vi "GOOPUtil Demo.vi"() -> ()   [LabVIEW 2012]
uses:
  <vilib>/addons/GOOPUtility/GOOPUtil_MemberDefinition.ctl
  <vilib>/addons/GOOPUtility/_Demo/GOOPUtil_Demo/AnotherClass_class/AnotherClass.lvclass
  <vilib>/addons/GOOPUtility/_Demo/GOOPUtil_Demo/DemoClass1_class/DemoClass1.lvclass
  <vilib>/addons/GOOPUtility/_Demo/GOOPUtil_Demo/DemoSubClass1_class/DemoSubClass1.lvclass
  <vilib>/addons/GOOPUtility/_Demo/GOOPUtil_Demo/DemoSubClass2_class/DemoSubClass2.lvclass
  <vilib>/addons/GOOPUtility/_Demo/GOOPUtil_Demo/DemoSubSubClass1_class/DemoSubSubClass1.lvclass
  <vilib>/addons/GOOPUtility/GOOPUtility.lvlib
panel:
  out "Class Path":path
  out "Another class constant IsEmpty?":bool
  out "AnotherClass constant Not a refnum?":bool
  out "Another Class Not a refnum?":bool
  out "Has AnotherClass SameAncestor DemoSubClass2?":bool
  out "Has DemoSubSubClass 1 SameAncestor DemoSubClass2?":bool
  out "Is DemoSubClass1 InstanceOf DemoSubClass2":bool
  out "Is DemoSubSubClass 1 InstanceOf DemoSubClass1?":bool
  out "Full Class Name":string
  out "lvlib Hierarchy":string[](array[string])
  out "Class Name":string
  out "IsCastReferenceEmpty?":bool
  out "IsLVObjectEmpty?":bool
  out "MemberPaths":T1[](array[typedef])
  out "Nr Of Killed Objects":i32
  out "error out":errorcluster
  in  "Destructor":enum16{"Generic Destroy", "Garbage Collector"}(ring)
  # "1. LV Object constant"
  # "2. DemoClass1 object"
  # "Doesn't work when\n.lvclass is inside an exe."
  # "3. DemoSubClass1 object"
  # "4. DemoSubSubClass object"
  # "5. DemoSubClass1 object"
  # "6. AnotherClass object"
  # "Notice: When building an application, the front panels of the Create(), Destroy() and GetObjectStatus()\nmustn't be removed. There is a trick to prevent them to be removed, by adding a \"dummy\"\ncontrol reference (or local variable) to the diagram somewhere, else you have to change the\nsettings in the build script for each of these VIs."
  # "7. AnotherClass constant"
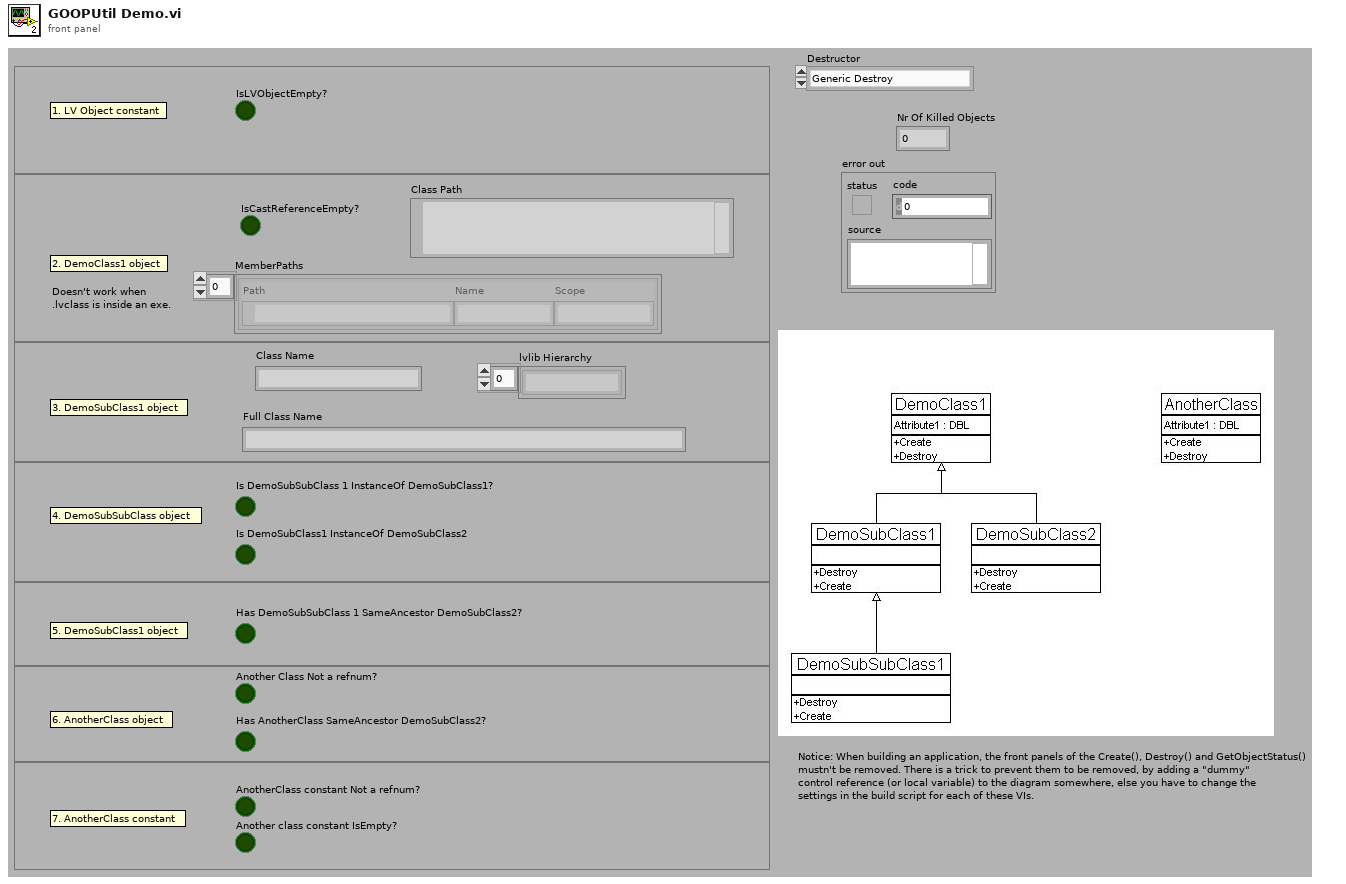
[diagram p1: front panel]
types:
  T1 = typedef "GOOPUtility.lvlib/GOOPUtil_MemberDefinition.ctl" = cluster{"Path":path, "Name":string, "Scope":string}
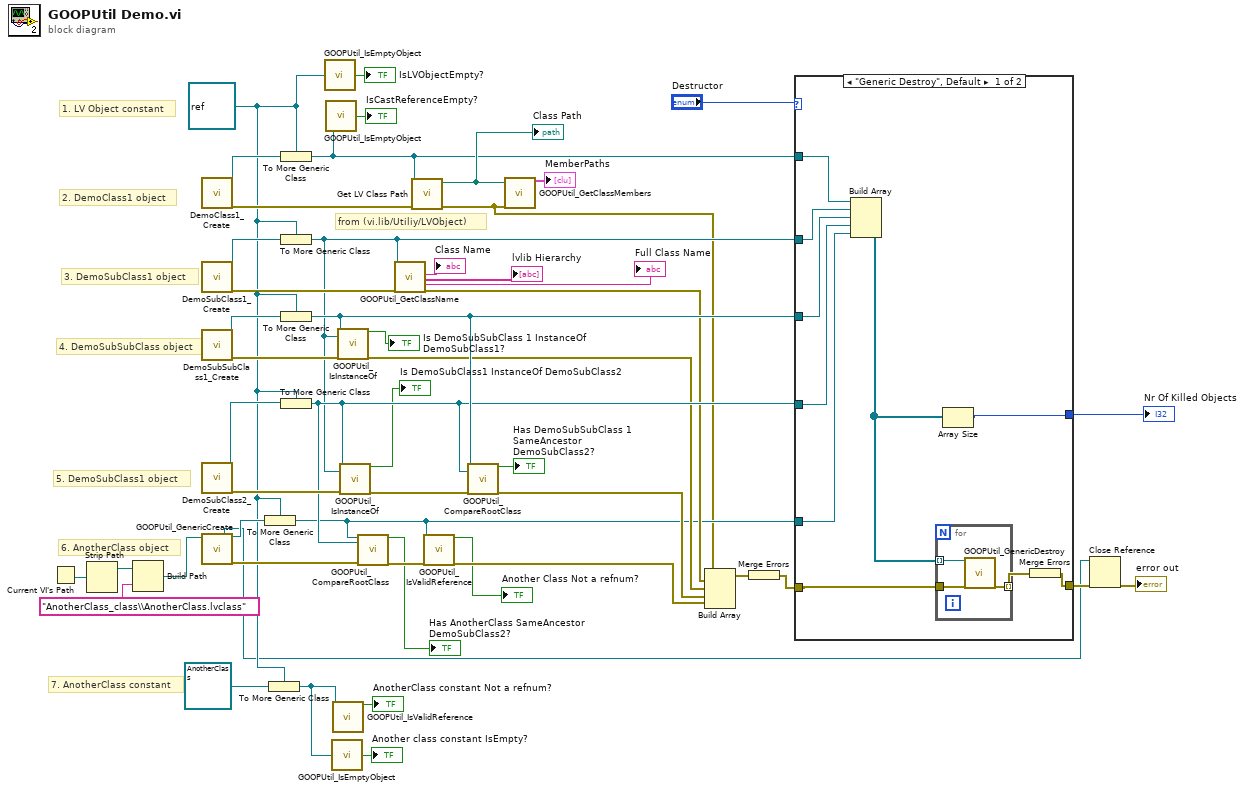
[diagram p0: block diagram]
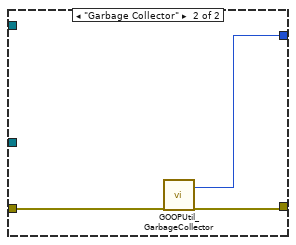
[diagram p2: hidden frame]
diagram:
  w26 = refnum<class> refnum ("LabVIEW Object")
  # "7. AnotherClass constant"
  # "6. AnotherClass object"
  # "5. DemoSubClass1 object"
  # "4. DemoSubSubClass object"
  # "3. DemoSubClass1 object"
  # "2. DemoClass1 object"
  # "1. LV Object constant"
  # "from (vi.lib/Utiliy/LVObject)"
  n1 = Current VI's Path() -> (path=w7:path)
  n2 = Strip Path(path=w7) -> (stripped path=w6:path)  [unwired: 1 out]
  n3 = Build Path(base path=w6, name or relative path="AnotherClass_class\\AnotherClass.lvclass") -> (appended path=w5:path)
  n4 = call <vilib>:"DemoClass1_Create.vi"() -> ("reference out"=w49:refnum<class "DemoClass1.lvclass">, "error out"=w41:errorcluster)  [unwired: 18 in]
  n5 = call <vilib>:"DemoSubClass1_Create.vi"() -> ("reference out"=w48:refnum<class "DemoSubClass1.lvclass">, "error out"=w32:errorcluster)  [unwired: 18 in]
  n6 = call <vilib>:"DemoSubSubClass1_Create.vi"() -> ("reference out"=w47:refnum<class "DemoSubSubClass1.lvclass">, "error out"=w37:errorcluster)  [unwired: 18 in]
  n7 = call <vilib>:"DemoSubClass2_Create.vi"() -> ("reference out"=w46:refnum<class "DemoSubClass2.lvclass">, "error out"=w38:errorcluster)  [unwired: 18 in]
  n8 = call <vilib>:"GOOPUtil_GenericCreate.vi"("GOOP Class Path"=w5) -> ("GOOP constructor VI ref"=w1:refnum<vi>, "GOOP Object"=w45:refnum<class>, "error out"=w36:errorcluster)  [unwired: 16 in]
  n9 = To More Generic Class(target class=w26, reference=w45) -> (generic class reference=w20:refnum<class>)
  n10 = To More Generic Class(target class=w26, reference=refnum<class "AnotherClass.lvclass"> refnum ("reference out")) -> (generic class reference=w21:refnum<class>)
  n11 = To More Generic Class(target class=w26, reference=w49) -> (generic class reference=w28:refnum<class>)
  n12 = To More Generic Class(target class=w26, reference=w48) -> (generic class reference=w30:refnum<class>)
  n13 = To More Generic Class(target class=w26, reference=w47) -> (generic class reference=w34:refnum<class>)
  n14 = To More Generic Class(target class=w26, reference=w46) -> (generic class reference=w33:refnum<class>)
  n15 = call <vilib>:"GOOPUtil_IsEmptyObject.vi"("LabVIEW Object"=w26) -> ("IsEmpty?"=→"IsLVObjectEmpty?":bool)
  n16 = call <vilib>:"GOOPUtil_IsEmptyObject.vi"("LabVIEW Object"=w28) -> ("IsEmpty?"=→"IsCastReferenceEmpty?":bool)
  n17 = call <vilib>:"GOOPUtil_IsEmptyObject.vi"("LabVIEW Object"=w21) -> ("IsEmpty?"=→"Another class constant IsEmpty?":bool)
  n18 = call <vilib>:"GOOPUtil_IsValidReference.vi"("LabVIEW Object"=w21) -> ("Not a refnum?"=→"AnotherClass constant Not a refnum?":bool)  [unwired: 16 in, 2 out]
  n19 = call <vilib>:"GOOPUtil_IsInstanceOf.vi"("GOOP Object"=w34, "Is Instance of Object"=w30, "error in (no error)"=w37) -> ("IsInstanceOf"=→"Is DemoSubSubClass 1 InstanceOf DemoSubClass1?":bool, "error out"=w24:errorcluster)  [unwired: 15 in]
  n20 = call <vilib>:"GOOPUtil_IsInstanceOf.vi"("GOOP Object"=w33, "Is Instance of Object"=w30, "error in (no error)"=w38) -> ("IsInstanceOf"=→"Is DemoSubClass1 InstanceOf DemoSubClass2":bool, "error out"=w35:errorcluster)  [unwired: 15 in]
  n21 = call <vilib>:"GOOPUtil_CompareRootClass.vi"("GOOP Object 1"=w20, "GOOP Object 2"=w33, "error in (no error)"=w36) -> ("SameAncestor"=→"Has AnotherClass SameAncestor DemoSubClass2?":bool, "error out"=w25:errorcluster)  [unwired: 13 in, 2 out]
  n22 = call <vilib>:"GOOPUtil_GetClassName.vi"("LabVIEW Object"=w30, "error in (no error)"=w32) -> ("Class Name"=→"Class Name":string, "lvlib Hierarchy"=→"lvlib Hierarchy":string[], "Full Class Name"=→"Full Class Name":string, "error out"=w31:errorcluster)  [unwired: 13 in, 1 out]
  n23 = call <vilib>:"Get LV Class Path.vi"("error in (no error)"=w41, "object"=w28) -> ("error out"=w8:errorcluster, "class path"=w40:path)  [unwired: 8 in]
  "Class Path" <- w40
  n24 = call <vilib>:"GOOPUtil_IsValidReference.vi"("LabVIEW Object"=w20, "error in (no error)"=w25) -> ("Not a refnum?"=→"Another Class Not a refnum?":bool, "error out"=w22:errorcluster)  [unwired: 15 in, 1 out]
  n25 = call <vilib>:"GOOPUtil_CompareRootClass.vi"("GOOP Object 1"=w34, "GOOP Object 2"=w33, "error in (no error)"=w35) -> ("SameAncestor"=→"Has DemoSubSubClass 1 SameAncestor DemoSubClass2?":bool, "error out"=w23:errorcluster)  [unwired: 13 in, 2 out]
  n26 = call <vilib>:"GOOPUtil_GetClassMembers.vi"("LVClassPath"=w40, "error in (no error)"=w8) -> ("MemberPaths"=→"MemberPaths":T1[])  [unwired: 16 in, 1 out]
  n27 = Build Array(w8, w31, w24, w23, w22) -> (w50:errorcluster[])
  n28 = Merge Errors(w50) -> (w44:errorcluster)
  n29 = case shown="\"Generic Destroy\", Default" "Destructor" {
    tunnel: w28 -> [w60 _]
    tunnel: w30 -> [w59 _]
    tunnel: w34 -> [w58 _]
    tunnel: w44 -> [w57 w66]
    tunnel: w33 -> [w56 _]
    tunnel: w20 -> [w55 _]
    tunnel: [w51 w65] -> w2
    tunnel: [w52 w64] -> w42
    frame "Generic Destroy", Default {
      n30 = Build Array(w60, w59, w58, w56, w55) -> (w53:refnum<class>[])
      n31 = for {
        tunnel: w57 -> [w63]
        tunnel: [w62] -> w54 mode=indexing
        tunnel: w53 -> [w61] mode=indexing
        n32 = call <vilib>:"GOOPUtil_GenericDestroy.vi"("GOOPObject"=w61, "error in (no error)"=w63) -> ("error out"=w62:errorcluster)  [unwired: 17 in]
      }
      n33 = Array Size(array=w53) -> (size(s)=w52:i32)
      n34 = Merge Errors(w54) -> (w51:errorcluster)
    }
    frame "Garbage Collector" {
      n35 = call <vilib>:"GOOPUtil_GarbageCollector.vi"("error in (no error)"=w66) -> ("Nr Of Killed Objects"=w64:i32, "error out"=w65:errorcluster)  [unwired: 17 in]
    }
  }
  "Nr Of Killed Objects" <- w42
  n36 = Close Reference(reference=w1, error in (no error)=w2) -> (error out=→"error out":errorcluster)
